vi "UMLEditor CommentsDialog.vi"(5 "error in (no error)":errorcluster) -> (15 "nameOut":string, 16 "commentsOut":string, 17 "canceled":bool, 19 "error out":errorcluster)   [LabVIEW 2012]
doc: "Helpinstructions."
panel:
  in  "Comment":string
  in  "Your name or e-mail":string
  in  "send":bool
  in  "cancel":bool
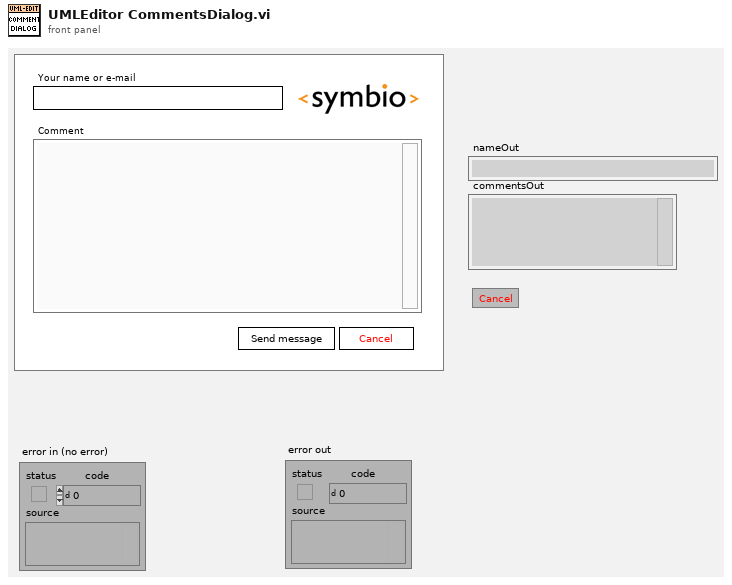
[diagram p1: front panel]
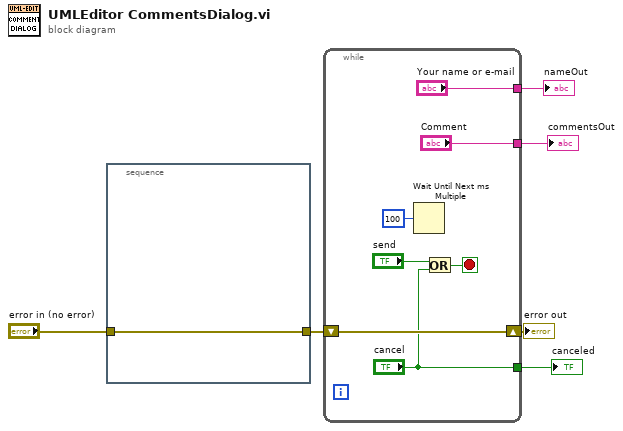
[diagram p0: block diagram]
diagram:
  n1 = stacked-sequence {
    tunnel: "error in (no error)" -> [w7]
    tunnel: [w7] -> w4
    frame #0 {
    }
  }
  n2 = while {
    shift-left: w4 -> [w13]
    shift-right: [w13] -> w6
    tunnel: ["Comment"] -> w3
    tunnel: ["Your name or e-mail"] -> w2
    tunnel: ["cancel"] -> w1
    stop <- w11 stop-if-true
    n3 = Wait Until Next ms Multiple(millisecond multiple=u32 100 ("milliseconds to wait")) -> ()  [unwired: 1 out]
    n4 = Or(x="send", y="cancel") -> (x .or. y?=w11:bool)
  }
  "error out" <- w6
  "commentsOut" <- w3
  "nameOut" <- w2
  "canceled" <- w1
